vi "Autonomous Independent.vi"   [LabVIEW 2016]
doc: "This VI is called when autonomous begins, and will automatically be terminated when autonomous ends. You can carry out timed or sensor driven robot movement independently without needing to return to the caller."
uses:
  <vilib>/Rock Robotics/WPI/SafetyOutput/WPI_SafetyOutputConfigMenu.ctl
  <vilib>/Rock Robotics/WPI/Utilities/WPI_GetSetVariantRefNum.vi
  <vilib>/Rock Robotics/Network Tables/NT Read String.vi
  <vilib>/Rock Robotics/WPI/Ultrasonic/WPI_SonarMB1010AnalogRefNum Registry Get.vi
  <vilib>/Rock Robotics/Network Tables/NT Read Number.vi
  <vilib>/Rock Robotics/WPI/Ultrasonic/WPI_SonarMB1010AnalogGetRange.vi
  <vilib>/Rock Robotics/WPI/RobotDrive/WPI_RobotDriveArcadeDrive_Standard(NoSaturation).vi
  <vilib>/Rock Robotics/Network Tables/NT Write Numeric Array.vi
types:
  T1 = typedef "WPI_JoystickDevRef.ctl" = cluster{"Device":T2}
  T2 = typedef "WPI_JoystickDeviceEnum.ctl" = enum16{"USB 0", "USB 1", "USB 2", "USB 3", "USB 4", "USB 5"}
  T3 = typedef "WPI_SafetyOutputConfigMenu.ctl" = enum16{"Enable", "Disable"}
  T4 = typedef "WPI_SonarMB1010AnalogDeviceRef.ctl" = cluster{"AIDeviceRef":T5, "Scaling factor (V/in)":dbl, "Average Bits":u8}
  T5 = typedef "WPI_AnalogChannelDevRef.ctl" = cluster{"DevStatus":errorcluster, "Analog Channel":T6}
  T6 = typedef "FPGA_AIChannel.ctl" = enum8{"AI 0", "AI 1", "AI 2", "AI 3", "AI MXP 0", "AI MXP 1", "AI MXP 2", "AI MXP 3", "Invalid"}
  T7 = typedef "WPI_RobotDriveDevRef.ctl" = cluster{"DevStatus":errorcluster, "Motors[]":T8[], "Square Inputs":bool, "Max Output":dbl}
  T8 = typedef "WPI_MotorControlDeviceRef.ctl" = cluster{"DeviceStatus":errorcluster, "Type":T9, "PWM":cluster{"PWM Channel":T10, "DeadBand":T11}, "CAN":cluster{"Device Number":u8, "SetOutput VI Ref":variant, "GetOutput VI Ref":variant, "Enable VI Ref":variant, "Disable VI Ref":variant, "Data":variant}, "Invert":bool}
  T9 = typedef "WPI_MotorControlType.ctl" = enum16{"PWM", "CAN"}
  T10 = typedef "FPGA_DIOPWMChannel.ctl" = enum8{"PWM 0", "PWM 1", "PWM 2", "PWM 3", "PWM 4", "PWM 5", "PWM 6", "PWM 7", "PWM 8", "PWM 9", "PWM MXP 0", "PWM MXP 1", "PWM MXP 2", "PWM MXP 3", "PWM MXP 4", "PWM MXP 5", "PWM MXP 6", "PWM MXP 7", "PWM MXP 8", "PWM MXP 9", "Invalid"}
  T11 = typedef "WPI_PWMDeadband.ctl" = cluster{"Name":string, "maxPositivePwm":i32, "minPositivePwm":i32, "centerPwm":i32, "maxNegativePwm":i32, "minNegativePwm":i32, "angularRange":u16}
  T12 = typedef "WPI_GyroDevRef.ctl" = cluster{"DevStatus":errorcluster, "Analog Channel":T6, "Offset":dbl, "Gain (VoltsPerDegree/Second)":dbl, "Gyro Type":enum16{"Analog", "XRS450"}, "Handle":i32, "SPI Bus":T13, "Device Found":bool, "Sample Rate":dbl, "Calibrate On Open":bool}
  T13 = typedef "spi_bus.ctl" = enum16{"SPI On-Board, CS0", "SPI On-Board, CS1", "SPI On-Board, CS2", "SPI On-Board, CS3", "SPI MXP", "Invalid"}
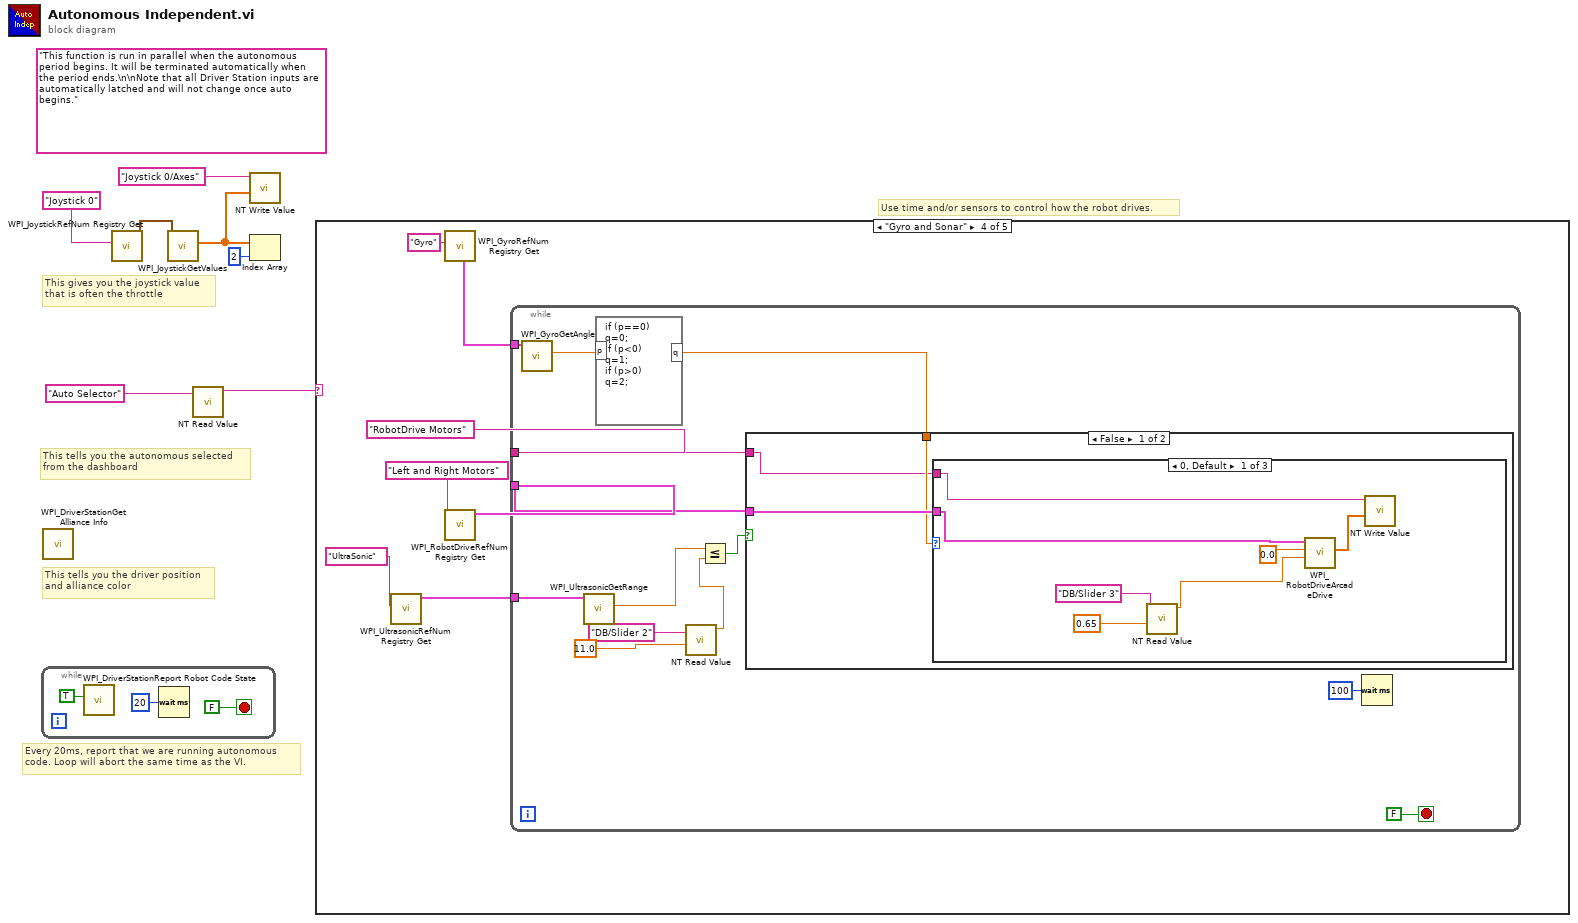
[diagram p0: block diagram]
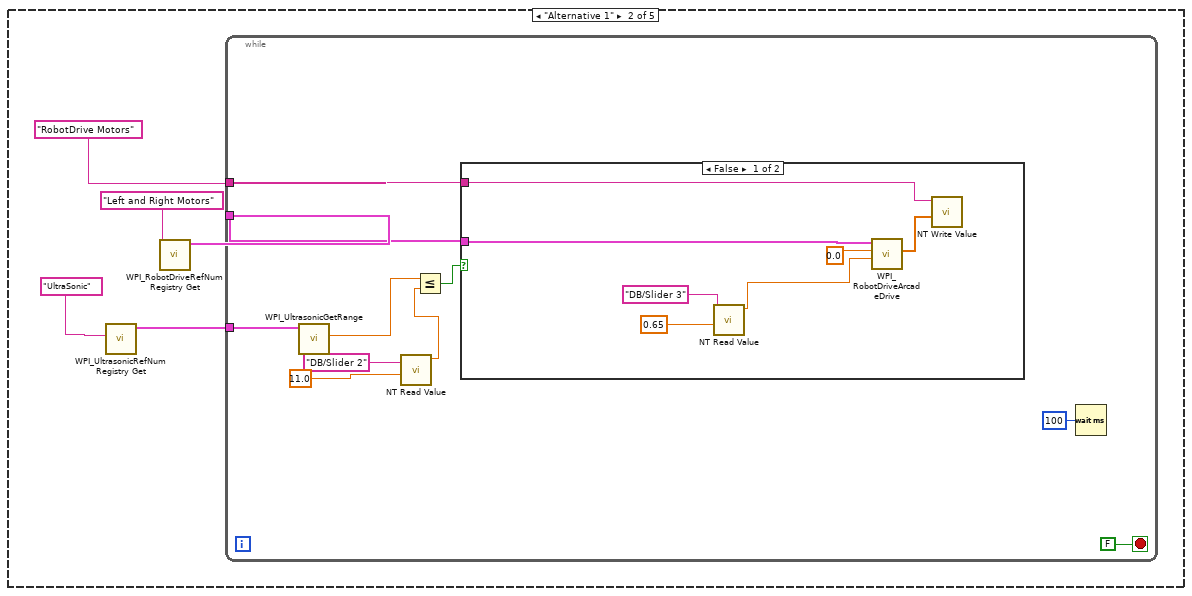
[diagram p3: hidden frame]
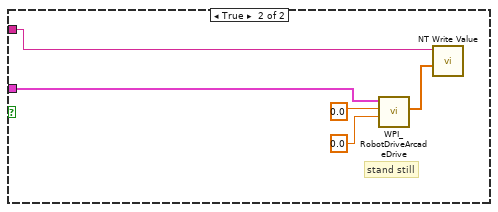
[diagram p4: hidden frame]
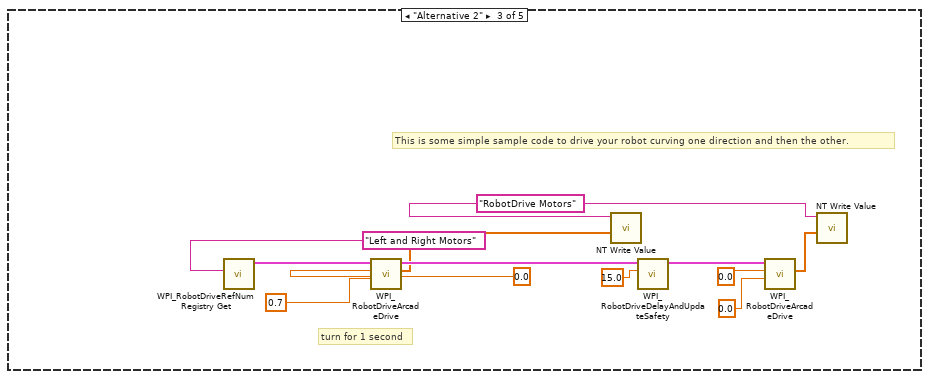
[diagram p5: hidden frame]
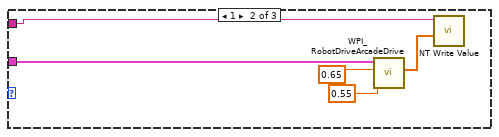
[diagram p6: hidden frame]
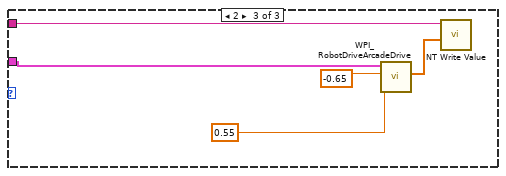
[diagram p7: hidden frame]
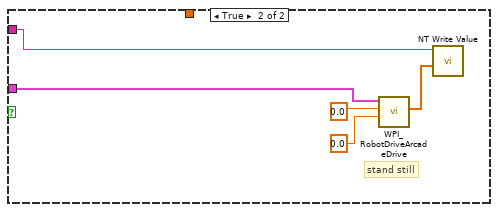
[diagram p8: hidden frame]
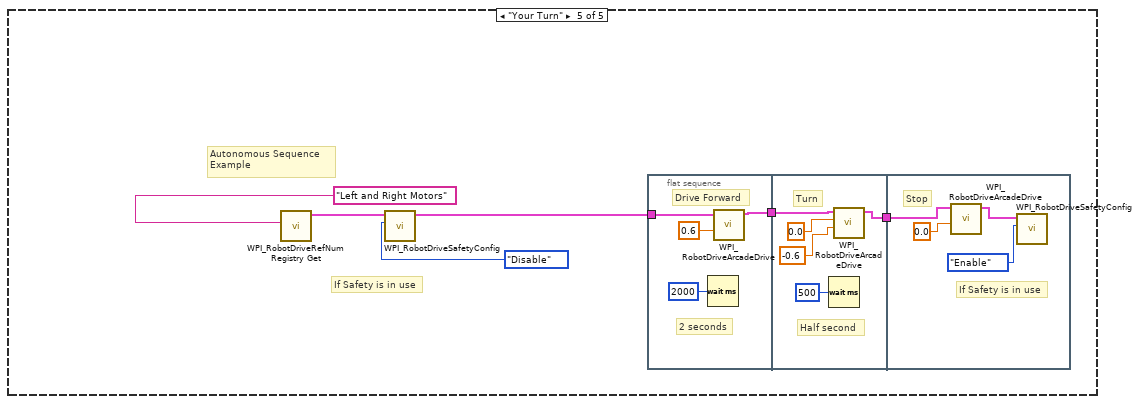
[diagram p9: hidden frame]
diagram:
  (unwired) "This function is run in parallel when the autonomous period begins. It will be terminated automatically when the period ends.\n\nNote that all Driver Station inputs are automatically latched and will not change once auto begins."
  # "This tells you the autonomous selected\nfrom the dashboard"
  # "Every 20ms, report that we are running autonomous\ncode. Loop will abort the same time as the VI."
  # "This gives you the joystick value\nthat is often the throttle"
  # "Use time and/or sensors to control how the robot drives."
  # "This tells you the driver position\nand alliance color"
  n1 = while {
    stop <- FALSE stop-if-true
    n2 = call <vilib>:"WPI_DriverStationReport Robot Code State.vi"("Autonomous"=TRUE) -> ()  [unwired: 10 in, 1 out]
    n3 = Wait (ms)(milliseconds to wait=u32 20) -> ()  [unwired: 1 out]
  }
  n4 = call <vilib>:"WPI_DriverStationGet Alliance Info.vi"() -> ()  [unwired: 12 out]
  n5 = call <vilib>:"WPI_JoystickRefNum Registry Get.vi"("refnum name"="Joystick 0") -> ("JoystickDevRef"=w6:T1)  [unwired: 1 in, 9 out]
  n6 = call <vilib>:"WPI_JoystickGetValues.vi"("JoystickDevRef"=w6) -> ("Axes"=w2:dbl[])  [unwired: 6 in, 4 out]
  n7 = call-poly <vilib>:"NT Read Value.vi"("Name"="Auto Selector") -> ("String"=w3:string)  [unwired: 9 in, 1 out]
  n8 = call-poly <vilib>:"NT Write Value.vi"("Numeric Array"=w2, "Name"="Joystick 0/Axes") -> ()  [unwired: 9 in, 1 out]
  n9 = Index Array(array=w2, index=2) -> ()  [unwired: 1 out]
  n10 = case shown="\"Gyro and Sonar\"" w3 {
    frame Default {
      # "You can put your main auto here, or you can right-click on the case and make any\nother frame be the default case."
      # "This is the frame that will execute if no selection is made, or if it is not recognized"
    }
    frame "Alternative 1" {
      n11 = call-poly <vilib>:"WPI_UltrasonicRefNum Registry Get.vi"("refnum name"="UltraSonic") -> ("SonarMB1010AnalogDevRef"=w11:T4)  [unwired: 9 in, 1 out]
      n12 = call <vilib>:"WPI_RobotDriveRefNum Registry Get.vi"("refnum name"="Left and Right Motors") -> ("RobotDriveDevRef"=w12:T7)  [unwired: 1 in, 9 out]
      n13 = while {
        tunnel: "RobotDrive Motors" ("Name") -> [w24]
        tunnel: w12 -> [w23]
        tunnel: w11 -> [w21]
        stop <- FALSE stop-if-true
        n14 = call-poly <vilib>:"WPI_UltrasonicGetRange.vi"("SonarMB1010AnalogDevRef"=w21) -> ("Distance"=w22:dbl)  [unwired: 8 in, 2 out]
        n15 = call-poly <vilib>:"NT Read Value.vi"("Default Value"=11.0 ("y"), "Name"="DB/Slider 2") -> ("Numeric"=w18:dbl)  [unwired: 8 in, 1 out]
        n16 = Less Or Equal?(x=w22, y=w18) -> (x <= y?=w25:bool)
        n17 = case shown="False" w25 {
          tunnel: w24 -> [w27 w33]
          tunnel: w23 -> [w26 w34]
          frame False {
            n18 = call-poly <vilib>:"NT Read Value.vi"("Default Value"=0.65, "Name"="DB/Slider 3") -> ("Numeric"=w30:dbl)  [unwired: 8 in, 1 out]
            n19 = call-poly <vilib>:"WPI_RobotDriveArcadeDrive.vi"("Y axis value"=w30, "X axis value"=0.0, "RobotDriveDevRef"=w26) -> ("Motor Values"=w29:dbl[])  [unwired: 1 in, 7 out]
            n20 = call-poly <vilib>:"NT Write Value.vi"("Numeric Array"=w29, "Name"=w27) -> ()  [unwired: 9 in, 1 out]
          }
          frame True {
            # "stand still"
            n21 = call-poly <vilib>:"WPI_RobotDriveArcadeDrive.vi"("Y axis value"=0.0 ("X axis value"), "X axis value"=0.0, "RobotDriveDevRef"=w34) -> ("Motor Values"=w37:dbl[])  [unwired: 1 in, 7 out]
            n22 = call-poly <vilib>:"NT Write Value.vi"("Numeric Array"=w37, "Name"=w33) -> ()  [unwired: 9 in, 1 out]
          }
        }
        n23 = Wait (ms)(milliseconds to wait=u32 100) -> ()  [unwired: 1 out]
      }
    }
    frame "Alternative 2" {
      w40 = "RobotDrive Motors" ("Name")
      # "This is some simple sample code to drive your robot curving one direction and then the other."
      # "turn for 1 second"
      n24 = call <vilib>:"WPI_RobotDriveRefNum Registry Get.vi"("refnum name"="Left and Right Motors") -> ("RobotDriveDevRef"=w49:T7)  [unwired: 1 in, 9 out]
      n25 = call-poly <vilib>:"WPI_RobotDriveArcadeDrive.vi"("Y axis value"=0.7 ("Default Value"), "X axis value"=0.0, "RobotDriveDevRef"=w49) -> ("Motor Values"=w39:dbl[], "RobotDriveDevRef"=w45:T7)  [unwired: 1 in, 6 out]
      n26 = call-poly <vilib>:"NT Write Value.vi"("Numeric Array"=w39, "Name"=w40) -> ()  [unwired: 9 in, 1 out]
      n27 = call <vilib>:"WPI_RobotDriveDelayAndUpdateSafety.vi"("Delay (s)"=15.0, "RobotDriveDevRef"=w45) -> ("RobotDriveDevRef 2"=w46:T7)  [unwired: 8 in, 1 out]
      n28 = call-poly <vilib>:"WPI_RobotDriveArcadeDrive.vi"("Y axis value"=0.0 ("X axis value"), "X axis value"=0.0, "RobotDriveDevRef"=w46) -> ("Motor Values"=w41:dbl[])  [unwired: 1 in, 7 out]
      n29 = call-poly <vilib>:"NT Write Value.vi"("Numeric Array"=w41, "Name"=w40) -> ()  [unwired: 9 in, 1 out]
    }
    frame "Gyro and Sonar" {
      n30 = call-poly <vilib>:"WPI_UltrasonicRefNum Registry Get.vi"("refnum name"="UltraSonic") -> ("SonarMB1010AnalogDevRef"=w53:T4)  [unwired: 9 in, 1 out]
      n31 = call <vilib>:"WPI_GyroRefNum Registry Get.vi"("refnum name"="Gyro") -> ("GyroDevRef"=w50:T12)  [unwired: 9 in, 1 out]
      n32 = call <vilib>:"WPI_RobotDriveRefNum Registry Get.vi"("refnum name"="Left and Right Motors") -> ("RobotDriveDevRef"=w54:T7)  [unwired: 1 in, 9 out]
      n33 = while {
        tunnel: "RobotDrive Motors" ("Name") -> [w68]
        tunnel: w54 -> [w67]
        tunnel: w53 -> [w65]
        tunnel: w50 -> [w59]
        stop <- FALSE stop-if-true
        n34 = call <vilib>:"WPI_GyroGetAngle.vi"("GyroDevRef"=w59) -> ("Angle"=w58:dbl)  [unwired: 6 in, 4 out]
        n35 = call-poly <vilib>:"WPI_UltrasonicGetRange.vi"("SonarMB1010AnalogDevRef"=w65) -> ("Distance"=w66:dbl)  [unwired: 8 in, 2 out]
        n36 = formula code="if (p==0)\nq=0;\nif (p<0)\nq=1;\nif (p>0)\nq=2;"("p"=w58) -> ("q"=w57:dbl)
        n37 = call-poly <vilib>:"NT Read Value.vi"("Default Value"=11.0 ("y"), "Name"="DB/Slider 2") -> ("Numeric"=w62:dbl)  [unwired: 8 in, 1 out]
        n38 = Less Or Equal?(x=w66, y=w62) -> (x <= y?=w69:bool)
        n39 = case shown="False" w69 {
          tunnel: w68 -> [w70 w90]
          tunnel: w67 -> [w72 w91]
          tunnel: w57 -> [w71 _]
          frame False {
            n40 = case shown="0, Default" w71 {
              tunnel: w72 -> [w74 w82 w87]
              tunnel: w70 -> [w73 w80 w85]
              frame 0, Default {
                n41 = call-poly <vilib>:"NT Read Value.vi"("Default Value"=0.65, "Name"="DB/Slider 3") -> ("Numeric"=w77:dbl)  [unwired: 8 in, 1 out]
                n42 = call-poly <vilib>:"WPI_RobotDriveArcadeDrive.vi"("Y axis value"=w77, "X axis value"=0.0, "RobotDriveDevRef"=w74) -> ("Motor Values"=w76:dbl[])  [unwired: 1 in, 7 out]
                n43 = call-poly <vilib>:"NT Write Value.vi"("Numeric Array"=w76, "Name"=w73) -> ()  [unwired: 9 in, 1 out]
              }
              frame 1 {
                n44 = call-poly <vilib>:"WPI_RobotDriveArcadeDrive.vi"("Y axis value"=0.55, "X axis value"=0.65, "RobotDriveDevRef"=w82) -> ("Motor Values"=w84:dbl[])  [unwired: 1 in, 7 out]
                n45 = call-poly <vilib>:"NT Write Value.vi"("Numeric Array"=w84, "Name"=w80) -> ()  [unwired: 9 in, 1 out]
              }
              frame 2 {
                n46 = call-poly <vilib>:"WPI_RobotDriveArcadeDrive.vi"("Y axis value"=0.55, "X axis value"=-0.65, "RobotDriveDevRef"=w87) -> ("Motor Values"=w89:dbl[])  [unwired: 1 in, 7 out]
                n47 = call-poly <vilib>:"NT Write Value.vi"("Numeric Array"=w89, "Name"=w85) -> ()  [unwired: 9 in, 1 out]
              }
            }
          }
          frame True {
            # "stand still"
            n48 = call-poly <vilib>:"WPI_RobotDriveArcadeDrive.vi"("Y axis value"=0.0 ("X axis value"), "X axis value"=0.0, "RobotDriveDevRef"=w91) -> ("Motor Values"=w94:dbl[])  [unwired: 1 in, 7 out]
            n49 = call-poly <vilib>:"NT Write Value.vi"("Numeric Array"=w94, "Name"=w90) -> ()  [unwired: 9 in, 1 out]
          }
        }
        n50 = Wait (ms)(milliseconds to wait=u32 100) -> ()  [unwired: 1 out]
      }
    }
    frame "Your Turn" {
      # "If Safety is in use"
      # "Autonomous Sequence\nExample"
      n51 = call <vilib>:"WPI_RobotDriveRefNum Registry Get.vi"("refnum name"="Left and Right Motors") -> ("RobotDriveDevRef"=w97:T7)  [unwired: 9 in, 1 out]
      n52 = call <vilib>:"WPI_RobotDriveSafetyConfig.vi"("mode"=WPI_SafetyOutputConfigMenu."Disable", "RobotDriveDevRef"=w97) -> ("RobotDriveDevRef"=w96:T7)  [unwired: 8 in, 1 out]
      n53 = flat-sequence {
        tunnel: w96 -> [w102]
        tunnel: [w101] -> w100
        tunnel: [w108] -> w99
        tunnel: w100 -> [w107]
        tunnel: w99 -> [w111]
        frame #0 {
          # "2 seconds"
          # "Drive Forward"
          n54 = Wait (ms)(milliseconds to wait=u32 2000) -> ()  [unwired: 1 out]
          n55 = call-poly <vilib>:"WPI_RobotDriveArcadeDrive.vi"("Y axis value"=0.6 ("Left axis value"), "RobotDriveDevRef"=w102) -> ("RobotDriveDevRef"=w101:T7)  [unwired: 7 in, 2 out]
        }
        frame #1 {
          # "Half second"
          # "Turn"
          n56 = Wait (ms)(milliseconds to wait=u32 500) -> ()  [unwired: 1 out]
          n57 = call-poly <vilib>:"WPI_RobotDriveArcadeDrive.vi"("Y axis value"=-0.6 ("Right axis value"), "X axis value"=0.0 ("Left axis value"), "RobotDriveDevRef"=w107) -> ("RobotDriveDevRef"=w108:T7)  [unwired: 6 in, 2 out]
        }
        frame #2 {
          # "If Safety is in use"
          # "Stop"
          n58 = call-poly <vilib>:"WPI_RobotDriveArcadeDrive.vi"("Y axis value"=0.0 ("Left axis value"), "RobotDriveDevRef"=w111) -> ("RobotDriveDevRef"=w110:T7)  [unwired: 7 in, 2 out]
          n59 = call <vilib>:"WPI_RobotDriveSafetyConfig.vi"("mode"=WPI_SafetyOutputConfigMenu."Enable", "RobotDriveDevRef"=w110) -> ()  [unwired: 8 in, 2 out]
        }
      }
    }
  }
